vi "formula_expression_node.vi"() -> ()   [LabVIEW 2019]
panel:
  in  "stop":bool
  out "output variable":dbl
  out "Numeric 2":dbl
  out "x+y":dbl
  in  "x":dbl
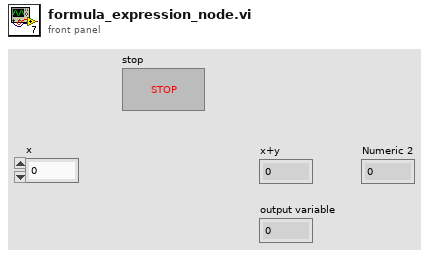
[diagram p1: front panel]
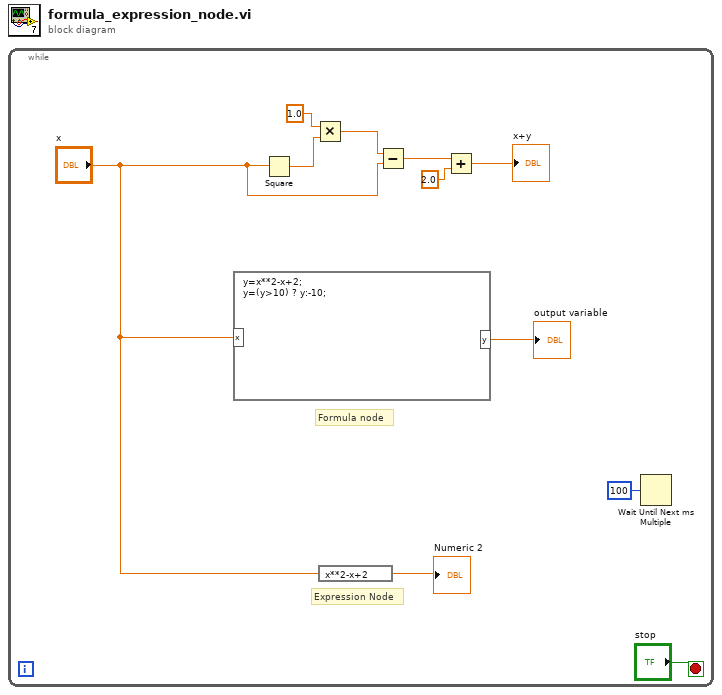
[diagram p0: block diagram]
diagram:
  n1 = while {
    stop <- "stop" stop-if-true
    # "Expression Node"
    # "Formula node"
    n2 = formula code="y=x**2-x+2;\ny=(y>10) ? y:-10;"("x"="x") -> ("y"=→"output variable":dbl)
    n3 = Square(x="x") -> (x^2=w6:dbl)
    n4 = Multiply(x=1.0, y=w6) -> (x*y=w8:dbl)
    n5 = expression code="x**2-x+2"("x") -> (→"Numeric 2":dbl)
    n6 = Subtract(x=w8, y="x") -> (x-y=w9:dbl)
    n7 = Add(x=w9, y=2.0) -> (x+y=→"x+y":dbl)
    n8 = Wait Until Next ms Multiple(millisecond multiple=u32 100) -> ()  [unwired: 1 out]
  }
